vi "Phasor Rotation due to Offset.vi"(6 "t0":ext, 9 "dt":ext, 10 "T":ext, 11 "j 2 pi f":cxt) -> (3 "exp(i 2 pi f theta_0)":cxt)   [LabVIEW 2021, in "Phasor.lvlib"]
uses:
  Phasor.lvlib
  e474b093-29b2-49b0-9b8d-466179359042.vi
  fabf79fc-6758-4714-a4ad-5851071bf14c.vi
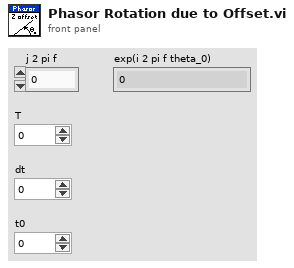
[diagram p1: front panel]
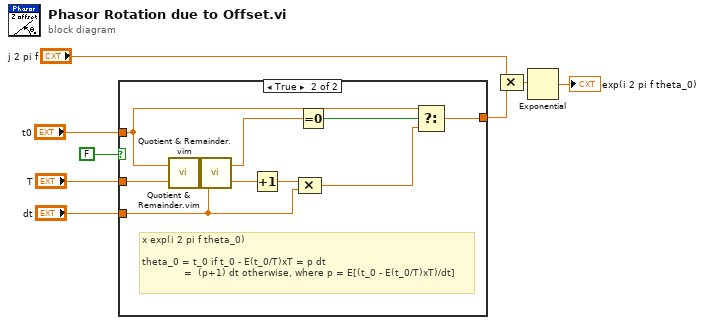
[diagram p0: block diagram]
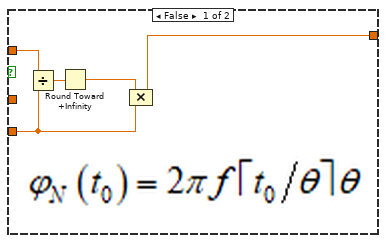
[diagram p2: hidden frame]
diagram:
  n1 = case shown="True" FALSE {
    tunnel: "dt" -> [w10 w14]
    tunnel: [w9 w20] -> w3
    tunnel: "t0" -> [w13 w18]
    tunnel: "T" -> [_ w15]
    frame False {
      n2 = Divide(x=w13, y=w10) -> (x/y=w12:ext)
      n3 = Round Toward +Infinity(x=w12) -> (ceil(x): smallest int >= x=w11:ext)
      n4 = Compound Arithmetic op=MULTIPLY(w11, w10) -> (w9:ext)
    }
    frame True {
      # "x exp(i 2 pi f theta_0)\n\ntheta_0 = t_0 if t_0 - E(t_0/T)xT = p dt\n              =  (p+1) dt otherwise, where p = E[(t_0 - E(t_0/T)xT)/dt]"
      n5 = call "Quotient & Remainder.vim"("y"=w15, "x"=w18) -> ("x - E(x/y)y"=w16:ext)  [unwired: 1 out]
      n6 = call "Quotient & Remainder.vim"("y"=w14, "x"=w16) -> ("E(x/y)"=w21:ext, "x - E(x/y)y"=w17:ext)
      n7 = Increment(x=w21) -> (x+1=w22:ext)
      n8 = Equal To 0?(x=w17) -> (x = 0?=w19:bool)
      n9 = Compound Arithmetic op=MULTIPLY(w22, w14) -> (w23:ext)
      n10 = Select(t=w18, s=w19, f=w23) -> (s? t:f=w20:ext)
    }
  }
  n11 = Compound Arithmetic op=MULTIPLY("j 2 pi f", w3) -> (w2:cxt)
  n12 = Exponential(1:w2) -> (0:→"exp(i 2 pi f theta_0)":cxt)
